vi "DownloadFile.vi"(5 "Path":path, 6 "error in":errorcluster, 9 "WebSocket connection":refnum<k5>) -> (0 "error out":errorcluster, 3 "WebSocket connection out":refnum<k5>)   [LabVIEW 2014, in "RasPiDownloader.lvlib"]
uses:
  RasPiDownloader.lvlib
  Websocket/Websocket.lvlib
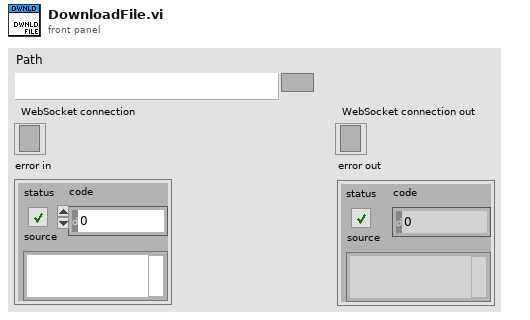
[diagram p1: front panel]
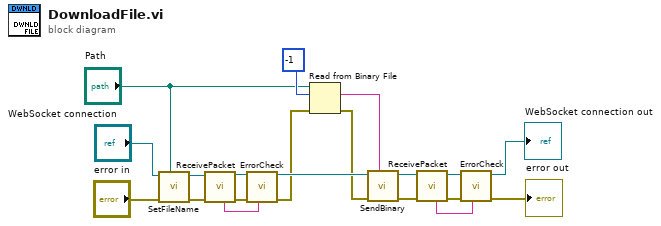
[diagram p0: block diagram]
diagram:
  n1 = call "SetFileName.vi"("Path"="Path", "error in"="error in", "WebSocket connection"="WebSocket connection") -> ("error out"=w18:errorcluster, "WebSocket connection out"=w17:refnum<k5>)  [unwired: 5 in]
  n2 = call "ReceivePacket.vi"("error in"=w18, "connection ID"=w17) -> ("error out"=w10:errorcluster, "connection ID out"=w15:refnum<k5>, "payload"=w7:string)  [unwired: 5 in]
  n3 = call "ErrorCheck.vi"("payload"=w7, "error in"=w10) -> ("error out"=w9:errorcluster)  [unwired: 7 in]
  n4 = Read from Binary File(8:w9, 10:-1 ("count (1)"), 11:"Path") -> (0:w14:errorcluster, 2:w13:string)  [unwired: 3 in, 2 out]
  n5 = call "SendBinary.vi"("payload"=w13, "error in"=w14, "connection ID"=w15) -> ("error out"=w12:errorcluster, "connection ID out"=w11:refnum<k5>)  [unwired: 5 in]
  n6 = call "ReceivePacket.vi"("error in"=w12, "connection ID"=w11) -> ("error out"=w8:errorcluster, "connection ID out"=→"WebSocket connection out":refnum<k5>, "payload"=w2:string)  [unwired: 5 in]
  n7 = call "ErrorCheck.vi"("payload"=w2, "error in"=w8) -> ("error out"=→"error out":errorcluster)  [unwired: 7 in]
